vi "Simple Session Test.vi"() -> ()   [LabVIEW 2020]
uses:
  G-Embedded-Python-Interpreter-Toolkit/G-Embedded-Python-Interpreter-Toolkit.lvlib
panel:
  out "error out":errorcluster
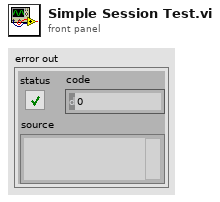
[diagram p1: front panel]
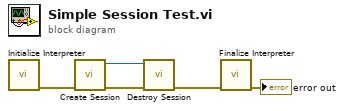
[diagram p0: block diagram]
diagram:
  n1 = call "Initialize Interpreter.vi"() -> ("error out"=w4:errorcluster)  [unwired: 10 in, 1 out]
  n2 = call "Create Session.vi"("error in (no error)"=w4) -> ("error out"=w5:errorcluster, "Session Handle"=w3:refnum<data-value>)  [unwired: 9 in]
  n3 = call "Destroy Session.vi"("error in (no error)"=w5, "Session Handle"=w3) -> ("error out"=w2:errorcluster)  [unwired: 9 in]
  n4 = call "Finalize Interpreter.vi"("error in (no error)"=w2) -> ("error out"=→"error out":errorcluster)  [unwired: 10 in]
